vi "GPSRMC.vi"(0 "String":string) -> (1 "Hora":string, 2 "Ubicación":string, 3 "Velocidad":string, 4 "Fecha":string)   [LabVIEW 2020]
doc: "Este programa desglosa las tramas rmc"
panel:
  out "A or V":string
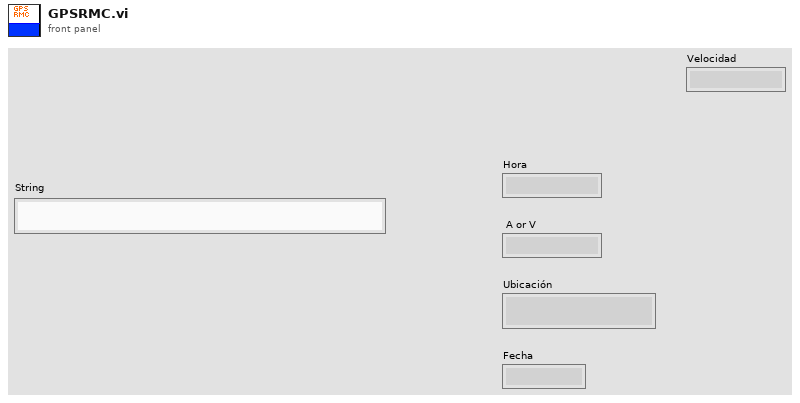
[diagram p1: front panel]
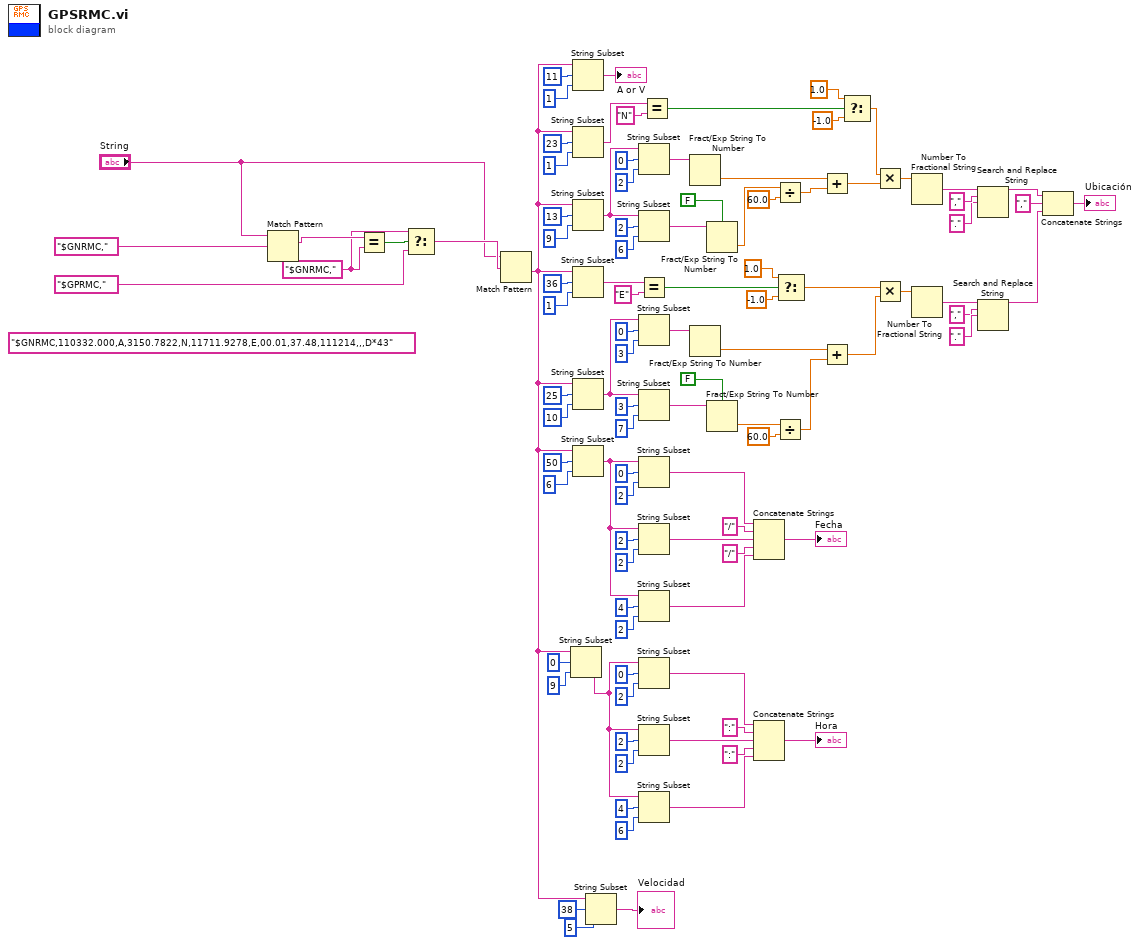
[diagram p0: block diagram]
diagram:
  w4 = "$GNRMC," ("regular expression")
  (unwired) "$GNRMC,110332.000,A,3150.7822,N,11711.9278,E,00.01,37.48,111214,,,D*43"
  n1 = Match Pattern(string="String", regular expression="$GNRMC,") -> (match substring=w6:string)  [unwired: 1 in, 3 out]
  n2 = Equal?(x=w6, y=w4) -> (x = y?=w5:bool)
  n3 = Select(t=w4, s=w5, f="$GPRMC," ("regular expression")) -> (s? t:f=w3:string)
  n4 = Match Pattern(string="String", regular expression=w3) -> (after substring=w11:string)  [unwired: 1 in, 3 out]
  n5 = String Subset(string=w11, offset (0)=0, length (rest)=9 ("length (rest)")) -> (substring=w36:string)
  n6 = String Subset(string=w11, offset (0)=11, length (rest)=1 ("length (rest)")) -> (substring=→"A or V":string)
  n7 = String Subset(string=w11, offset (0)=23, length (rest)=1 ("length (rest)")) -> (substring=w81:string)
  n8 = String Subset(string=w11, offset (0)=13, length (rest)=9 ("length (rest)")) -> (substring=w93:string)
  n9 = String Subset(string=w11, offset (0)=36, length (rest)=1 ("length (rest)")) -> (substring=w55:string)
  n10 = String Subset(string=w11, offset (0)=25, length (rest)=10 ("length (rest)")) -> (substring=w65:string)
  n11 = String Subset(string=w11, offset (0)=50, length (rest)=6 ("length (rest)")) -> (substring=w20:string)
  n12 = String Subset(string=w11, offset (0)=38, length (rest)=5 ("length (rest)")) -> (substring=→"Velocidad":string)
  n13 = String Subset(string=w93, offset (0)=0, length (rest)=2 ("length (rest)")) -> (substring=w89:string)
  n14 = String Subset(string=w93, offset (0)=2, length (rest)=6 ("length (rest)")) -> (substring=w90:string)
  n15 = Equal?(x=w55, y="E") -> (x = y?=w57:bool)
  n16 = String Subset(string=w65, offset (0)=0, length (rest)=3 ("length (rest)")) -> (substring=w69:string)
  n17 = String Subset(string=w65, offset (0)=3, length (rest)=7 ("length (rest)")) -> (substring=w68:string)
  n18 = String Subset(string=w20, offset (0)=0, length (rest)=2 ("length (rest)")) -> (substring=w17:string)
  n19 = String Subset(string=w20, offset (0)=2, length (rest)=2 ("length (rest)")) -> (substring=w15:string)
  n20 = String Subset(string=w20, offset (0)=4, length (rest)=2 ("length (rest)")) -> (substring=w13:string)
  n21 = String Subset(string=w36, offset (0)=0, length (rest)=2 ("length (rest)")) -> (substring=w33:string)
  n22 = String Subset(string=w36, offset (0)=2, length (rest)=2 ("length (rest)")) -> (substring=w31:string)
  n23 = String Subset(string=w36, offset (0)=4, length (rest)=6 ("length (rest)")) -> (substring=w29:string)
  n24 = Equal?(x=w81, y="N") -> (x = y?=w79:bool)
  n25 = Fract/Exp String To Number(string=w89) -> (number=w85:dbl)  [unwired: 3 in, 1 out]
  n26 = Fract/Exp String To Number(string=w69) -> (number=w73:dbl)  [unwired: 3 in, 1 out]
  n27 = Fract/Exp String To Number(use system decimal point (T)=FALSE, string=w90) -> (number=w87:dbl)  [unwired: 2 in, 1 out]
  n28 = Fract/Exp String To Number(use system decimal point (T)=FALSE, string=w68) -> (number=w71:dbl)  [unwired: 2 in, 1 out]
  n29 = Concatenate Strings(w17, "/" ("string"), w15, "/" ("string"), w13) -> (→"Fecha":string)
  n30 = Concatenate Strings(w33, ":" ("string"), w31, ":" ("string"), w29) -> (→"Hora":string)
  n31 = Divide(x=w87, y=60.0) -> (x/y=w84:dbl)
  n32 = Divide(x=w71, y=60.0) -> (x/y=w74:dbl)
  n33 = Select(t=1.0, s=w57, f=-1.0) -> (s? t:f=w60:dbl)
  n34 = Add(x=w85, y=w84) -> (x+y=w75:dbl)
  n35 = Add(x=w73, y=w74) -> (x+y=w54:dbl)
  n36 = Select(t=1.0, s=w79, f=-1.0) -> (s? t:f=w76:dbl)
  n37 = Multiply(x=w76, y=w75) -> (x*y=w51:dbl)
  n38 = Multiply(x=w60, y=w54) -> (x*y=w50:dbl)
  n39 = Number To Fractional String(number=w51) -> (F-format string=w49:string)  [unwired: 3 in]
  n40 = Number To Fractional String(number=w50) -> (F-format string=w44:string)  [unwired: 3 in]
  n41 = Search and Replace String(input string=w49, search string=",", replace string="." ("replace string (\"\")")) -> (result string=w41:string)  [unwired: 5 in, 3 out]
  n42 = Search and Replace String(input string=w44, search string=",", replace string="." ("replace string (\"\")")) -> (result string=w43:string)  [unwired: 5 in, 3 out]
  n43 = Concatenate Strings(w41, "," ("string"), w43) -> (→"Ubicación":string)
